vi "Zdrift_subVi.vi"(8 "error in (no error)":errorcluster, 10 "Duration":dbl, 11 "Application in":refnum<vi>) -> (0 "error out":errorcluster, 2 "z drift":dbl, 3 "Application out":refnum<vi>)   [LabVIEW 2014]
uses:
  <userlib>/Nanonis Prog Interface V5/Nanonis Prog Interface.lvlib
  <vilib>/Analysis/NI_AALPro.lvlib
panel:
  out "slope (m/s)":dbl format="%#_4p"
  out "elasped":dbl
  out "progress":u8(slide) scale=0.0..100.0
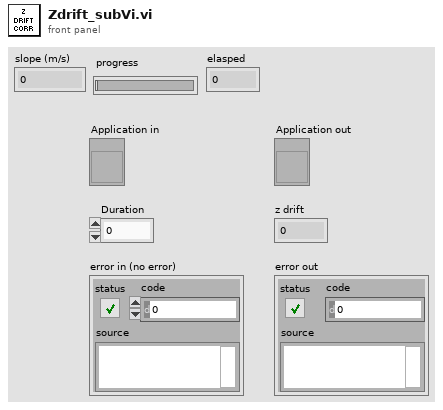
[diagram p1: front panel]
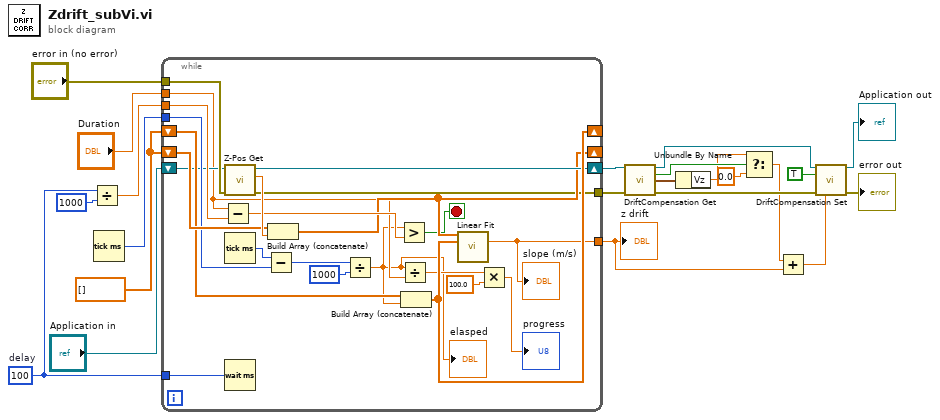
[diagram p0: block diagram]
diagram:
  w12 = u32 100  # delay
  w11 = sgl[] [] ("Array")
  n1 = Divide(x=w12, y=u32 1000) -> (x/y=w14:dbl)
  n2 = Tick Count (ms)() -> (millisecond timer value=w10:u32)
  n3 = while {
    tunnel: "error in (no error)" -> [w45]
    shift-right: [w31] -> _
    shift-left: w11 -> [w43]
    shift-right: [w34] -> _
    shift-left: w11 -> [w42]
    tunnel: w10 -> [w41]
    tunnel: w12 -> [w36]
    tunnel: w14 -> [w35]
    shift-right: [w32] -> w15
    shift-left: "Application in" -> [w33]
    tunnel: [w29] -> w16
    tunnel: "Duration" -> [w26]
    tunnel: [w28] -> w20
    stop <- w30 stop-if-true
    n4 = Subtract(x=w26, y=w35) -> (x-y=w37:dbl)
    n5 = call <userlib>:"Z-Pos Get.vi"("error in (no error)"=w45, "Application ref in"=w33) -> ("error out"=w29:errorcluster, "Z position (m)"=w44:sgl, "Application ref out"=w32:refnum<vi>)  [unwired: 7 in]
    n6 = Tick Count (ms)() -> (millisecond timer value=w38:u32)
    n7 = Wait (ms)(milliseconds to wait=w36) -> ()  [unwired: 1 out]
    n8 = Subtract(x=w38, y=w41) -> (x-y=w39:u32)
    n9 = Build Array (concatenate)(w43, w44) -> (w31:sgl[])
    n10 = Divide(x=w39, y=u32 1000) -> (x/y=w23:dbl)
    "elasped" <- w23
    n11 = Greater?(x=w23, y=w37) -> (0:w30:bool)
    n12 = Divide(x=w23, y=w26) -> (x/y=w27:dbl)
    n13 = Build Array (concatenate)(w42, w23) -> (w34:dbl[])
    n14 = call <vilib>:"Linear Fit.vi"("Y"=w31, "X"=w34) -> ("slope"=w28:dbl)  [unwired: 9 in, 4 out]
    "slope (m/s)" <- w28
    n15 = Multiply(x=w27, y=100.0) -> (x*y=→"progress":dbl)
  }
  "z drift" <- w20
  n16 = call <userlib>:"DriftCompensation Get.vi"("Application ref in"=w15, "error in (no error)"=w16) -> ("Application ref out"=w1:refnum<vi>, "Compensation status"=w7:bool, "Compensation speeds (m/s)"=w6:cluster{"Vx":sgl, "Vy":sgl, "Vz":sgl}, "error out"=w8:errorcluster)  [unwired: 9 in, 1 out]
  n17 = Unbundle By Name(w6) -> ("Vz"=w5:sgl)
  n18 = Select(t=w5, s=w7, f=sgl 0.0) -> (s? t:f=w3:sgl)
  n19 = Add(x=w3, y=w20) -> (x+y=w2:dbl)
  n20 = call <userlib>:"DriftCompensation Set.vi"("Application ref in"=w1, "Compensation On/Off"=TRUE, "error in (no error)"=w8, "Vz (m/s)"=w2) -> ("Application ref out"=→"Application out":refnum<vi>, "error out"=→"error out":errorcluster)  [unwired: 10 in]
